vi "SaveRefs.vi"(9 "All Refs Array Refnum":refnum<vi>, 10 "Array of label refnums":refnum<vi>[](array[refnum]), 11 "Path to refs":path=path "Z:/Programmes en Developpement/octo-labview/Turning Box PI Near Field/Moteurs PI/PI Refs") -> (0 "error out":errorcluster)   [LabVIEW 2014]
panel:
  in  "RefLabels 4":string(combo)
  in  "RefLabels 3":string(combo)
  in  "RefLabels 2":string(combo)
  in  "RefLabels 1":string(combo)
  in  "All refs":dbl[][](array[numeric]) format="%.6f"
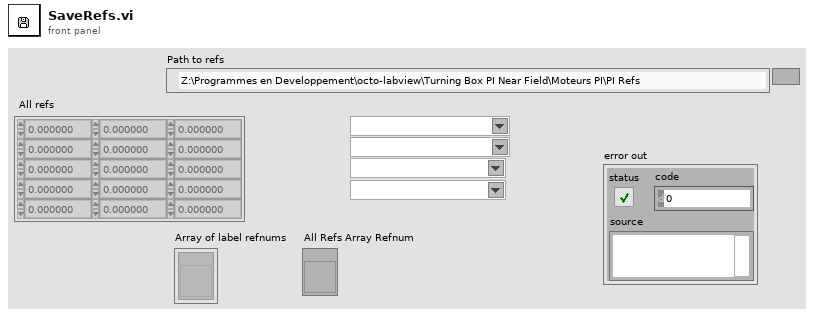
[diagram p1: front panel]
types:
  T1 = enum16{"open", "replace", "create", "open or create", "replace or create", "replace or create with confirmation"}
  T2 = typedef "LVComboBoxStrsAndValuesArrayTypeDef.ctl" = cluster{"String":string, "Value":string}[]
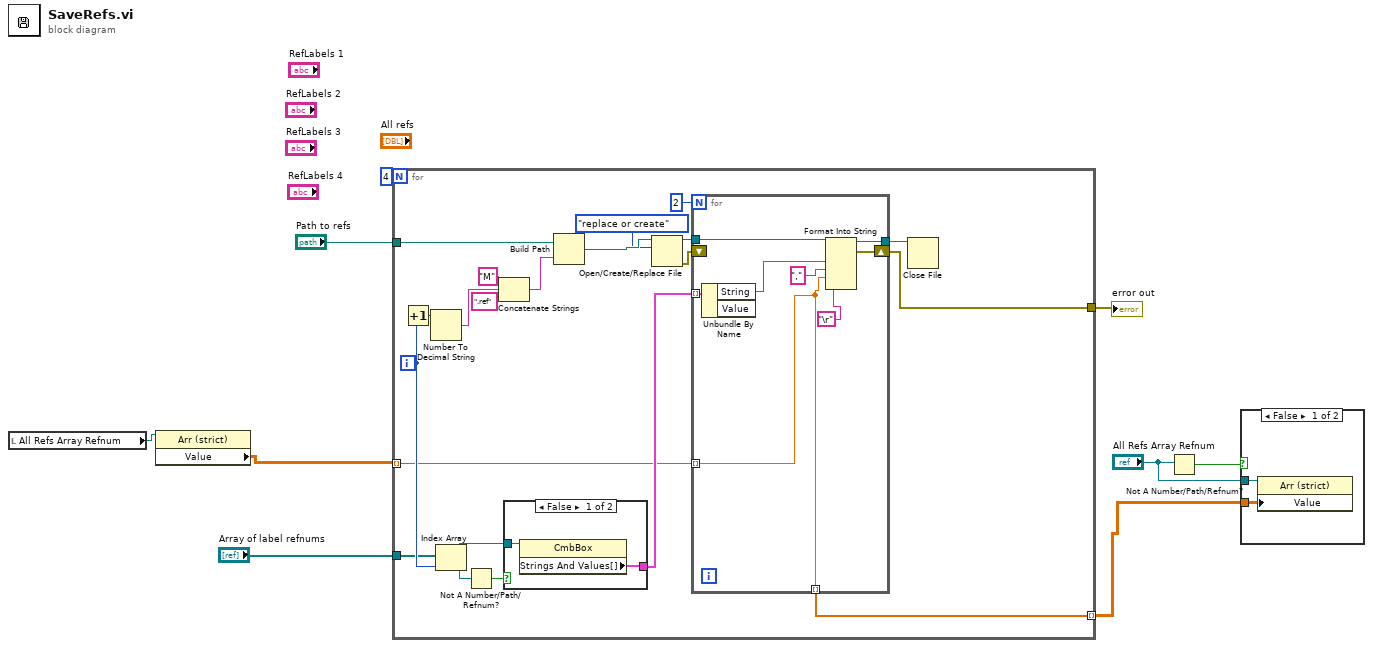
[diagram p0: block diagram]
diagram:
  n1 = local read "All Refs Array Refnum"() -> (w3:refnum<vi>)
  n2 = property class="Arr (strict)"(reference=w3) -> ("Value"=w1:dbl[][])  [unwired: 1 in, 2 out]
  n3 = for {
    N: 4 -> [_]
    tunnel: "Path to refs" -> [w29]
    tunnel: [w23] -> w2 mode=indexing
    tunnel: [w22] -> w7
    tunnel: "Array of label refnums" -> [w19]
    tunnel: w1 -> [w10] mode=indexing
    i -> [w20]
    n4 = Increment(x=w20) -> (x+1=w26:i32)
    n5 = Number To Decimal String(number=w26) -> (decimal integer string=w25:string)  [unwired: 1 in]
    n6 = Index Array(array=w19, index=w20) -> (element=w18:refnum<vi>)
    n7 = Not A Number/Path/Refnum?(number/path/refnum=w18) -> (NaN/Path/Refnum?=w21:bool)
    n8 = Concatenate Strings("M", w25, ".ref") -> (w24:string)
    n9 = case shown="False" w21 {
      tunnel: w18 -> [w39 _]
      tunnel: [w38 _] -> w11
      frame False {
        n10 = property class="CmbBox"(reference=w39) -> ("Strings And Values[]"=w38:T2)  [unwired: 1 in, 2 out]
      }
      frame True {
      }
    }
    n11 = Build Path(base path=w29, name or relative path=w24) -> (appended path=w17:path)
    n12 = Open/Create/Replace File(file path (use dialog)=w17, operation (0:open)=T1."replace or create") -> (refnum out=w16:refnum<file>, error out=w15:errorcluster)  [unwired: 4 in, 1 out]
    n13 = for {
      N: 2 -> [_]
      tunnel: w16 -> [w37]
      tunnel: [w36] -> w12
      tunnel: [w30] -> w23 mode=indexing
      shift-right: [w34] -> w22
      shift-left: w15 -> [_]
      tunnel: w11 -> [w32] mode=indexing
      tunnel: w10 -> [w30] mode=indexing
      n14 = Unbundle By Name(w32) -> ("String"=w31:string)  [unwired: 1 out]
      n15 = Format Into String(initial string=w37, w31, ",", w30, "\r") -> (resulting string=w36:refnum<file>, error out=w34:errorcluster)  [unwired: 2 in]
    }
    n16 = Close File(refnum=w12) -> ()  [unwired: 1 in, 2 out]
  }
  "error out" <- w7
  n17 = Not A Number/Path/Refnum?(number/path/refnum="All Refs Array Refnum") -> (NaN/Path/Refnum?=w6:bool)
  n18 = case shown="False" w6 {
    tunnel: w2 -> [w41 _]
    tunnel: "All Refs Array Refnum" -> [w40 _]
    frame False {
      n19 = property class="Arr (strict)"(reference=w40, "Value"=w41) -> ()  [unwired: 1 in, 2 out]
    }
    frame True {
    }
  }
